vi "FGV_RefTerminal.vi"(7 "Action":enum16{"Set Ref", "Get Ref"}(ring), 10 "refin":refnum<vi>) -> (2 "refout":refnum<vi>)   [LabVIEW 2014]
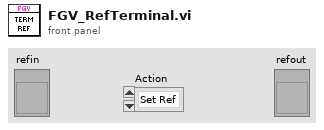
[diagram p1: front panel]
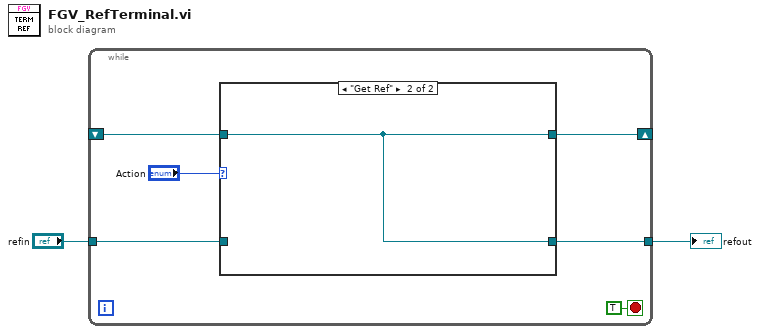
[diagram p0: block diagram]
diagram:
  n1 = while {
    tunnel: "refin" -> [w6]
    shift-right: [w5] -> _
    shift-left: _ -> [w3]
    tunnel: [w4] -> w1
    stop <- TRUE stop-if-true
    n2 = case shown="\"Get Ref\"" "Action" {
      tunnel: w6 -> [w9 _]
      tunnel: [w9 w10] -> w5
      tunnel: [_ w10] -> w4
      tunnel: w3 -> [_ w10]
      frame "Set Ref", Default {
      }
      frame "Get Ref" {
      }
    }
  }
  "refout" <- w1
